vi "温度压力采集.vi"() -> ()   [LabVIEW 2014]
panel:
  out "当前压力":dbl
  out "压力表":dbl(knob) scale=0.0..130.0
  out "实时压力显示":dbl(graph)
  out "最低压力":dbl
  out "平均压力":dbl
  out "最高压力":dbl
  out "当前温度":dbl
  out "实时温度显示":dbl(graph)
  out "温度计":dbl(slide) scale=0.0..100.0
  out "最高温度":dbl
  out "平均温度":dbl
  out "最低温度":dbl
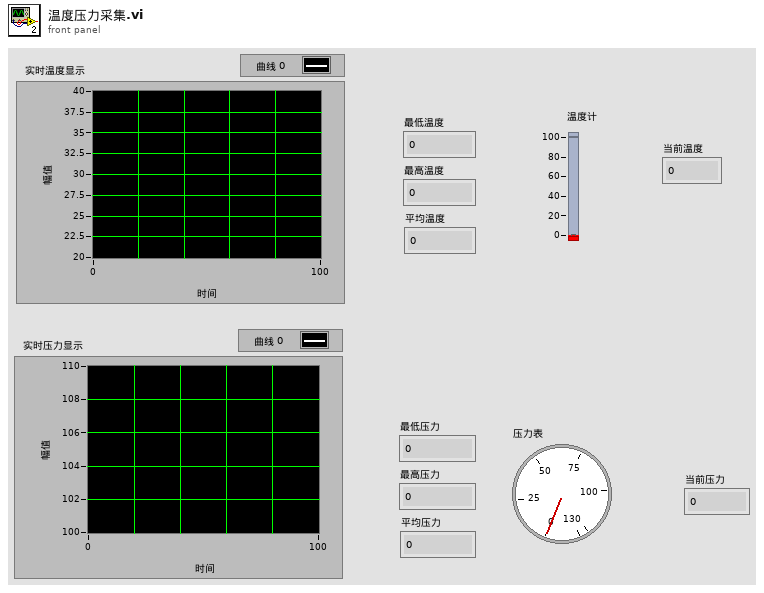
[diagram p1: front panel]
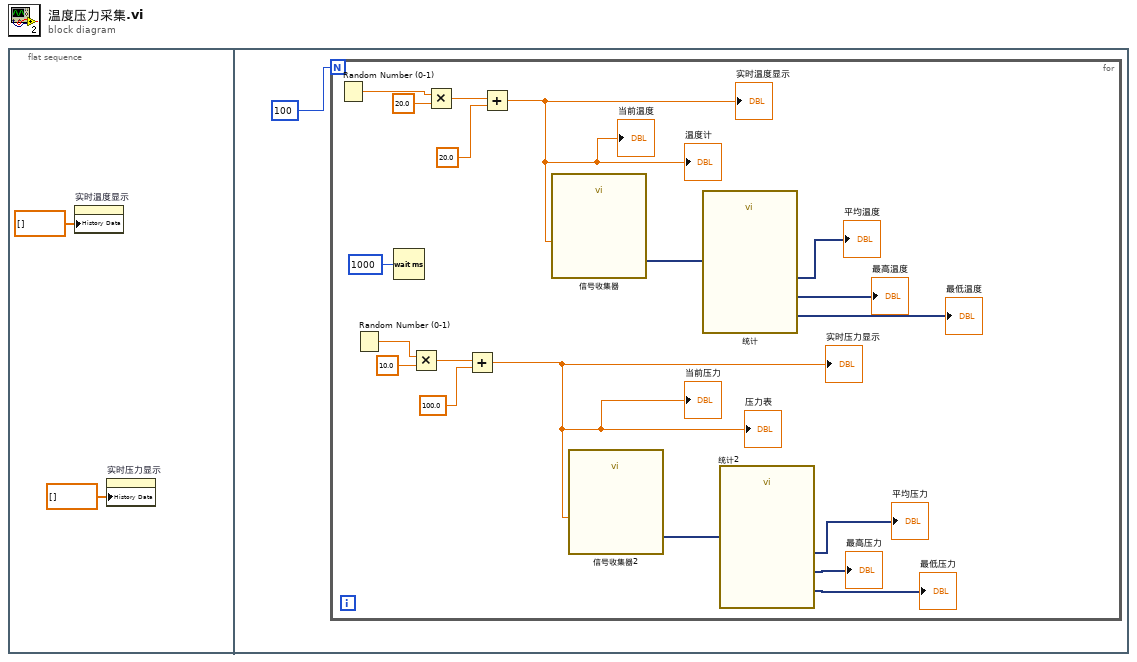
[diagram p0: block diagram]
diagram:
  n1 = flat-sequence {
    frame #0 {
      n2 = property on="实时温度显示" class="WFChart (严格)"("History Data"=dbl[] [] ("历史数据")) -> ()  [unwired: 2 in, 2 out]
      n3 = property on="实时压力显示" class="WFChart (严格)"("History Data"=dbl[] [] ("历史数据")) -> ()  [unwired: 2 in, 2 out]
    }
    frame #1 {
      n4 = for {
        N: 100 -> [_]
        n5 = Random Number (0-1)() -> (number: 0 to 1=w20:dbl)
        n6 = Random Number (0-1)() -> (number: 0 to 1=w12:dbl)
        n7 = Wait (ms)(milliseconds to wait=u32 1000 ("等待时间（毫秒）")) -> ()  [unwired: 1 out]
        n8 = Multiply(x=w12, y=10.0) -> (x*y=w11:dbl)
        n9 = Multiply(x=w20, y=20.0) -> (x*y=w19:dbl)
        n10 = Add(x=w11, y=100.0) -> (x+y=w5:dbl)
        "实时压力显示" <- w5
        "压力表" <- w5
        "当前压力" <- w5
        n11 = Add(x=w19, y=20.0) -> (x+y=w14:dbl)
        "温度计" <- w14
        "实时温度显示" <- w14
        "当前温度" <- w14
        n12 = call "信号收集器"("Signals"=w14) -> ("Collected Signals"=w17:dynamicdata)  [unwired: 9 in, 1 out]
        n13 = call "信号收集器2"("Signals"=w5) -> ("Collected Signals"=w9:dynamicdata)  [unwired: 9 in, 1 out]
        n14 = call "统计"("Signals"=w17) -> ("Arithmetic Mean"=→"平均温度":dynamicdata, "Minimum"=→"最低温度":dynamicdata, "Maximum"=→"最高温度":dynamicdata)  [unwired: 23 in, 1 out]
        n15 = call "统计2"("Signals"=w9) -> ("Arithmetic Mean"=→"平均压力":dynamicdata, "Minimum"=→"最低压力":dynamicdata, "Maximum"=→"最高压力":dynamicdata)  [unwired: 23 in, 1 out]
      }
    }
  }
